vi "Save Cfg File.vi"(8 "error in (no error)":errorcluster, 11 "[V] Sys Cfg Base in":refnum<class "[V] Sys Cfg Base.lvclass">) -> (0 "error out":errorcluster, 3 "[V] Sys Cfg Base out":refnum<class "[V] Sys Cfg Base.lvclass">)   [LabVIEW 2023, in "[V] Sys Cfg Base.lvlib" / "[V] Sys Cfg Base.lvclass"]
uses:
  [V] Sys Cfg Base.lvclass
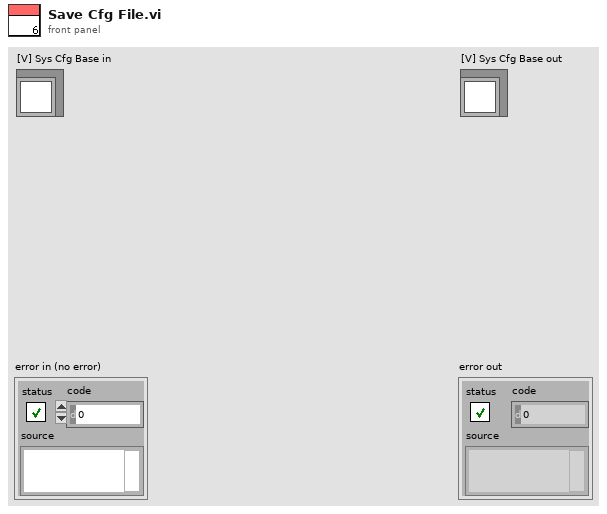
[diagram p1: front panel]
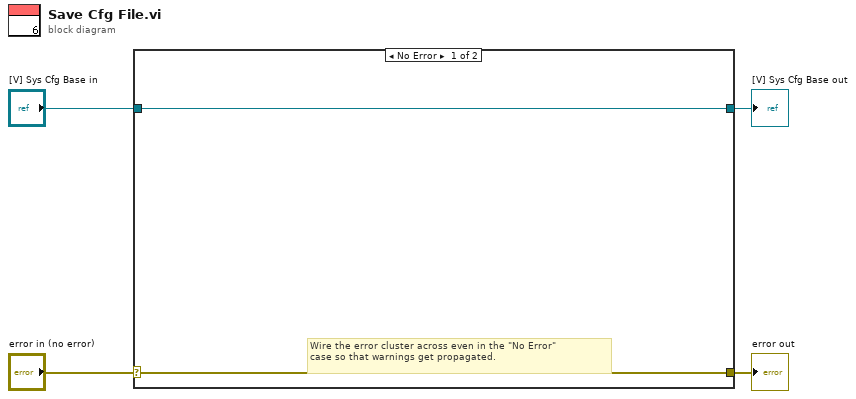
[diagram p0: block diagram]
diagram:
  n1 = case shown="No Error" "error in (no error)" {
    selector: "error in (no error)" -> [w5 w8]
    tunnel: [w5 w8] -> w3
    tunnel: [w6 w7] -> w1
    tunnel: "[V] Sys Cfg Base in" -> [w6 w7]
    frame No Error {
      # "Wire the error cluster across even in the \"No Error\"\ncase so that warnings get propagated."
    }
    frame Error {
    }
  }
  "error out" <- w3
  "[V] Sys Cfg Base out" <- w1
